vi "Update LC Line.vi"(1 "LC Stop":bool, 2 "LC Hold":bool) -> ()   [LabVIEW 2018]
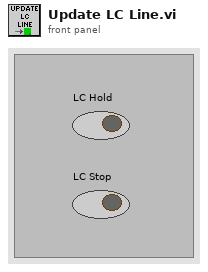
[diagram p1: front panel]
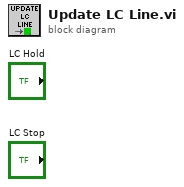
[diagram p0: block diagram]
diagram:
